vi "Process.vi"(8 "error in":errorcluster, 11 "Example Instrument UI":refnum<class "Instrument.Example UI.lvclass">) -> (0 "error out":errorcluster, 3 "Example Instrument UI out":refnum<class "Instrument.Example UI.lvclass">)   [LabVIEW 2016, in "Instrument.Example UI.lvclass"]
doc: "---------------------------------------------------------------\nJKI State Machine Objects™\nhttp://jki.net/state-machine-objects/\nCopyright (C) 2005-2015, JKI <info@jki.net>\nALL RIGHTS RESERVEDJKI State Machine Objects (SMO) 1.0.0.5\nJKI - JKI\nCopyright (c) 2016, JKI"
uses:
  Instrument.Example UI.lvclass
  C:/Program Files (x86)/National Instruments/LabVIEW 2016/vi.lib/JKI/JKI SMO/SMO/SMO.lvclass
  C:/Program Files (x86)/National Instruments/LabVIEW 2016/vi.lib/JKI/JKI SMO/SMO.UI/SMO.UI.lvclass
  <vilib>/JKI/JKI SMO/SMO/Typedefs/Parent Call--Enum.ctl
  Instrument.Example UI.lvclass/Instrument.Example UI.ctl
  <vilib>/JKI/JKI SMO/SMO.UI/SMO.UI.lvclass
  <vilib>/JKI/JKI SMO/SMO/SMO.lvclass
  <userlib>/LevyLab/Levylab Instruments/SMOs/Instrument/Instrument.lvclass
panel:
  in  "setConfig":bool
  in  "update time (ms)":u32=200
  in  "STOP":bool
  # "#todo\nmake UI here. maybe include a nice picture of the hardware?\n#todo\nadd buttons to do stuff (e.g., change a setting)\nButtons should trigger an event\n#todo\nresize this box if you want your UI to be different size"
  # "#todo\nthis control is refresh rate"
  # "SMO UI Template"
  # "For instructions on how to use the JKI State Machine Objects, examples and video tutorials, visit:\nhttp://jki.net/state-machine-objects/\n\nJKI State Machine Objects™\nhttp://jki.net/state-machine-objects/\nCopyright (C) 2005-2015, JKI <info@jki.net>\nALL RIGHTS RESERVED"
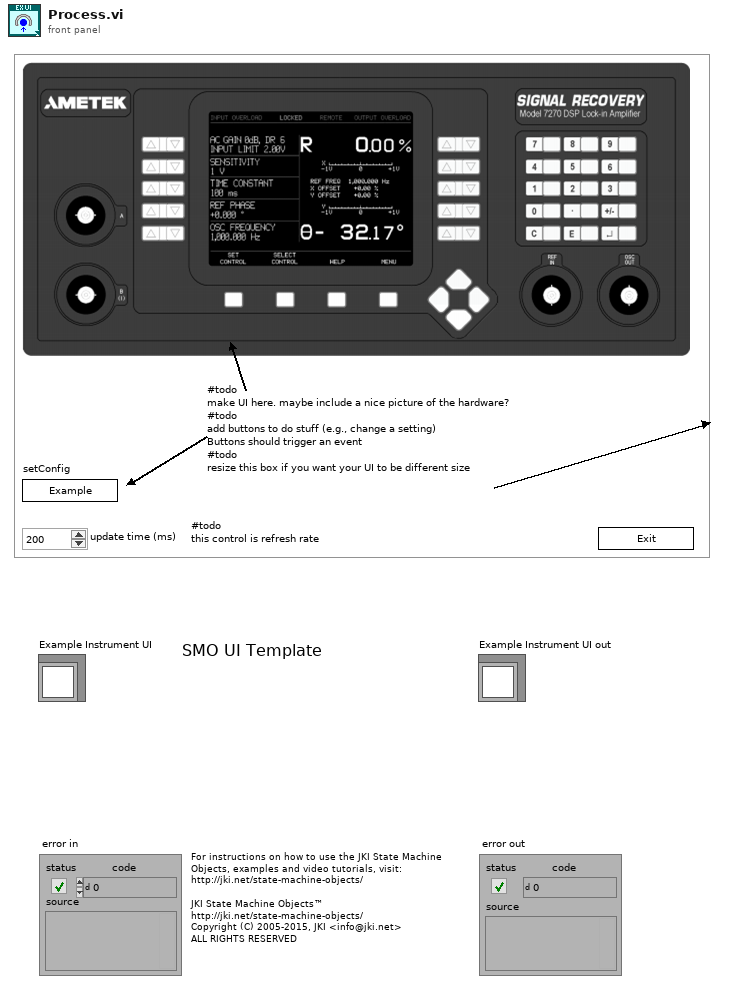
[diagram p1: front panel]
types:
  T1 = typedef "SMO.lvclass/Parent Call--Enum.ctl" = enum16{"Allows parent to run", "Does not request parent to run"}
  T2 = enum32{"invalid app kind", "Development System", "Run Time System", "Student Edition", "Embedded LabVIEW", "Evaluation", "Custom"}
  T3 = enum32{"Invalid", "Standard", "Closed", "Hidden", "Minimized", "Maximized"}
  T4 = cluster{"Core":cluster{"Current VI Reference":refnum<vi>, "Close Panel on Exit?":bool, "error":errorcluster}, "Self Reference":refnum<class "Instrument.Example UI.lvclass">, "Instrument":refnum<class "Instrument.lvclass">, "getAll":variant, "getDisplay":variant, "config":variant}
  T5 = cluster{"Current VI Reference":refnum<vi>, "Close Panel on Exit?":bool, "error":errorcluster}
  T6 = typedef "SMO.lvclass/Protected Events.ctl" = cluster{"StopProcesses":refnum<user-event>, "AbortProcesses":refnum<user-event>, "Config Changed":refnum<user-event>, "Dependency":refnum<user-event>}
  T7 = typedef "Instrument.lvclass/PublicEvents--Cluster.ctl" = cluster{"MessageFromProcess":refnum<user-event>}
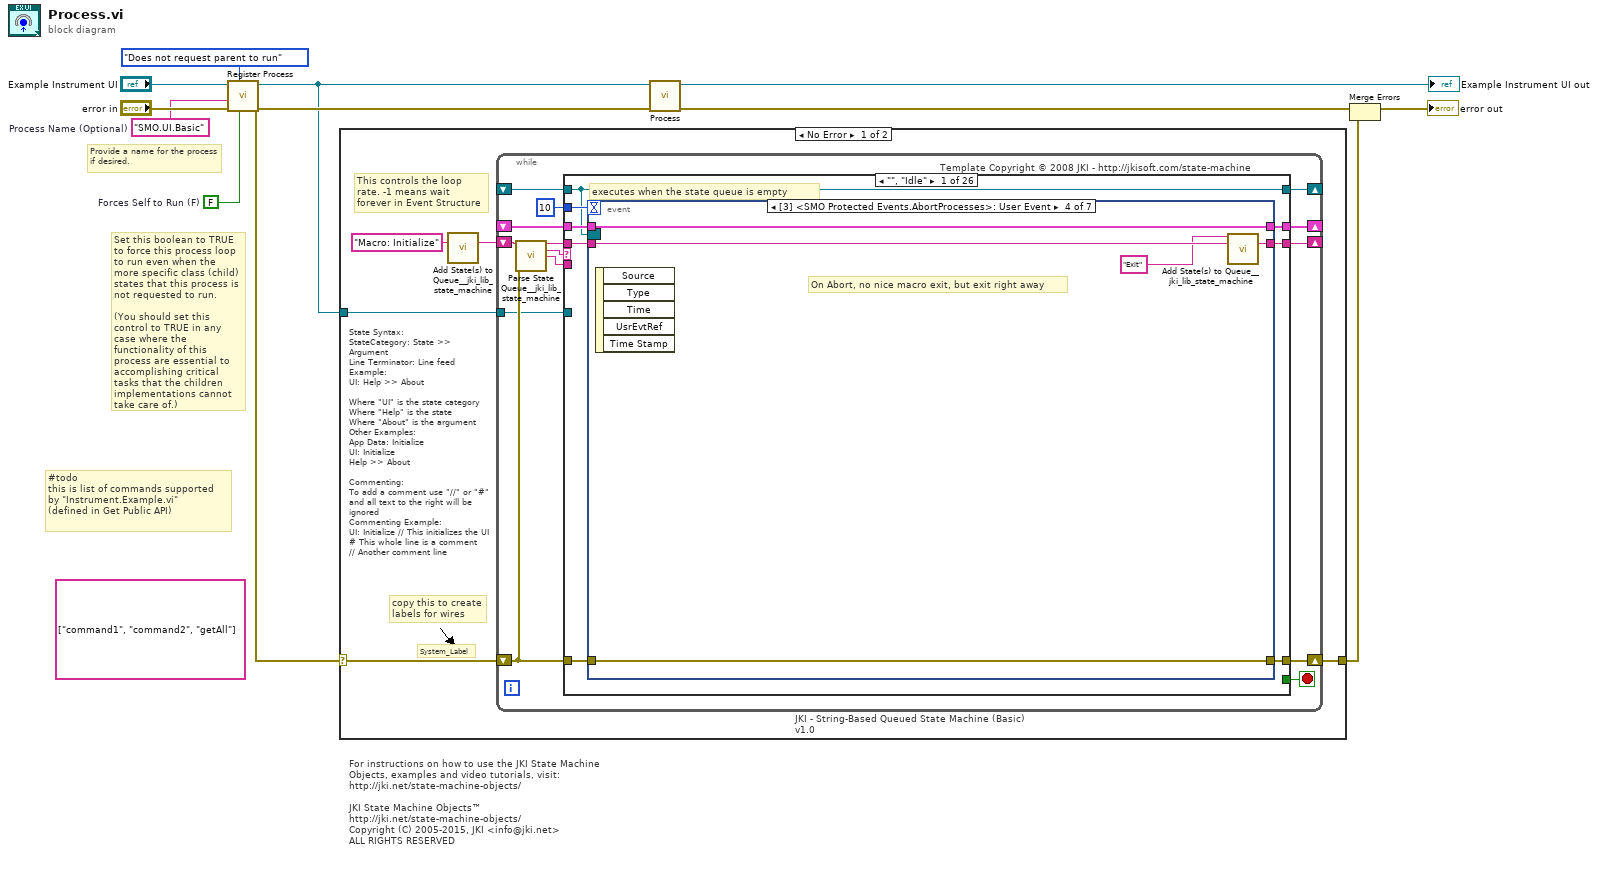
[diagram p0: block diagram]
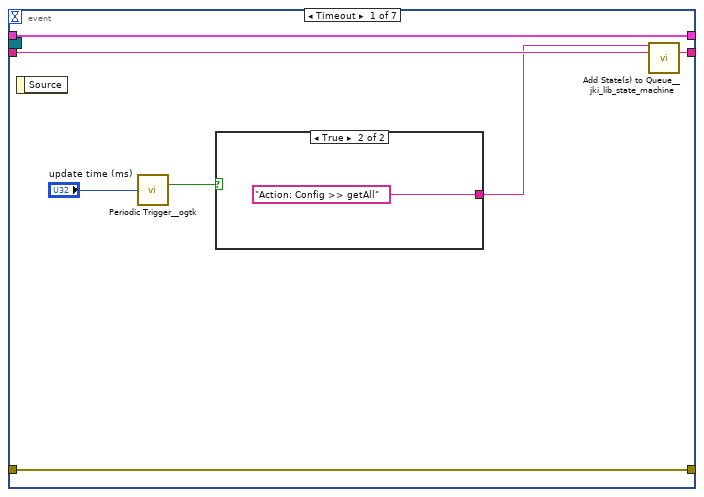
[diagram p2: hidden frame]
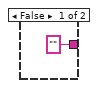
[diagram p3: hidden frame]
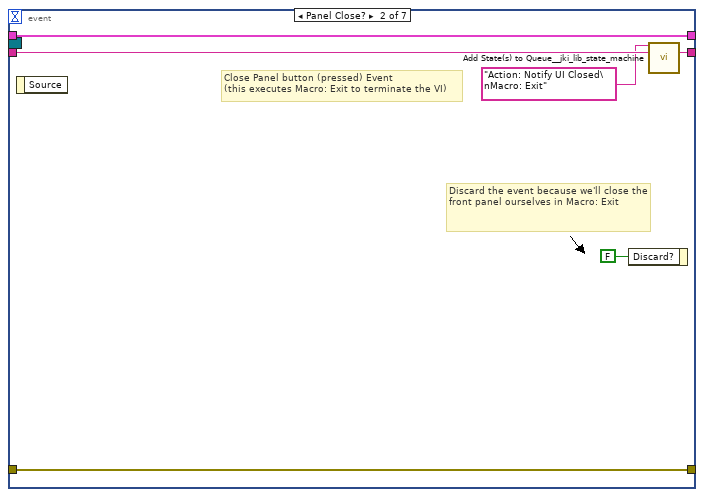
[diagram p4: hidden frame]
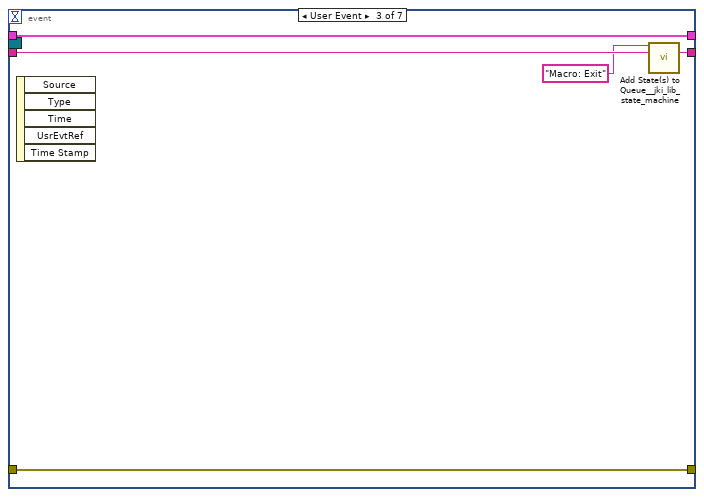
[diagram p5: hidden frame]
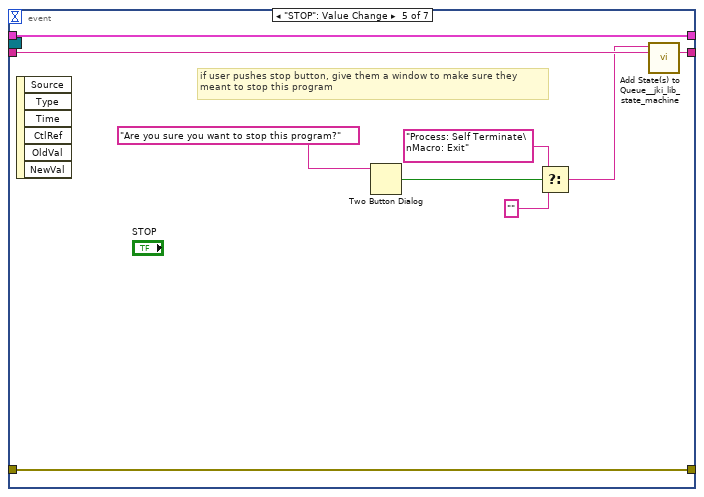
[diagram p6: hidden frame]
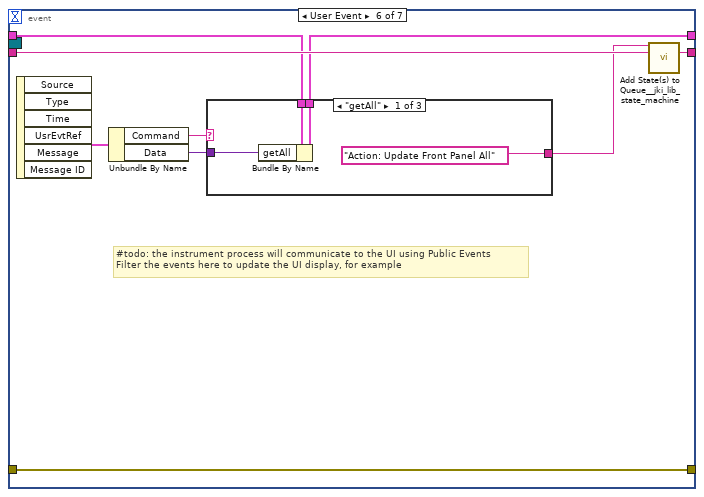
[diagram p7: hidden frame]
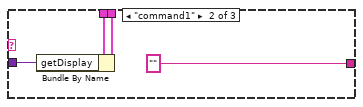
[diagram p8: hidden frame]
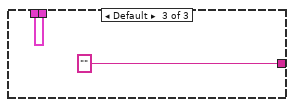
[diagram p9: hidden frame]
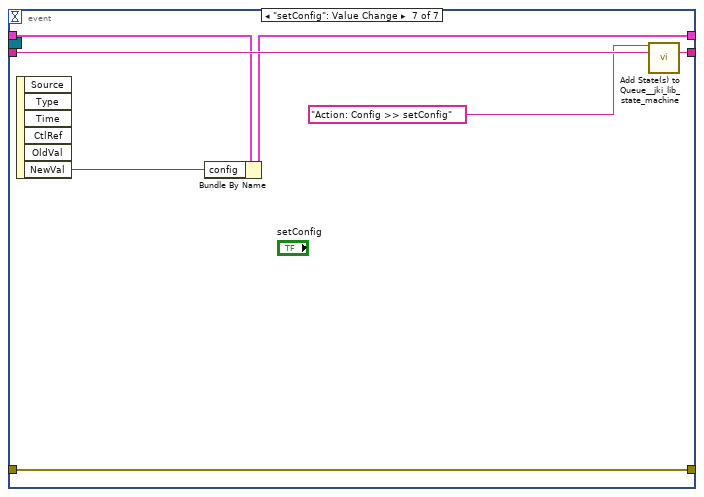
[diagram p10: hidden frame]
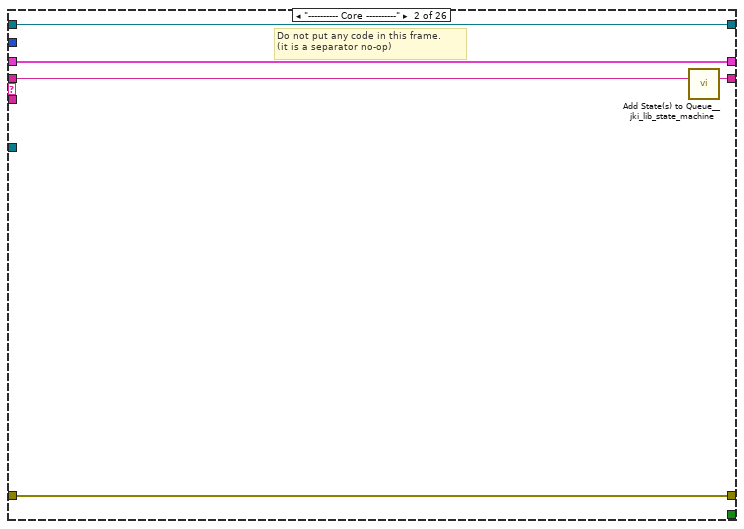
[diagram p11: hidden frame]
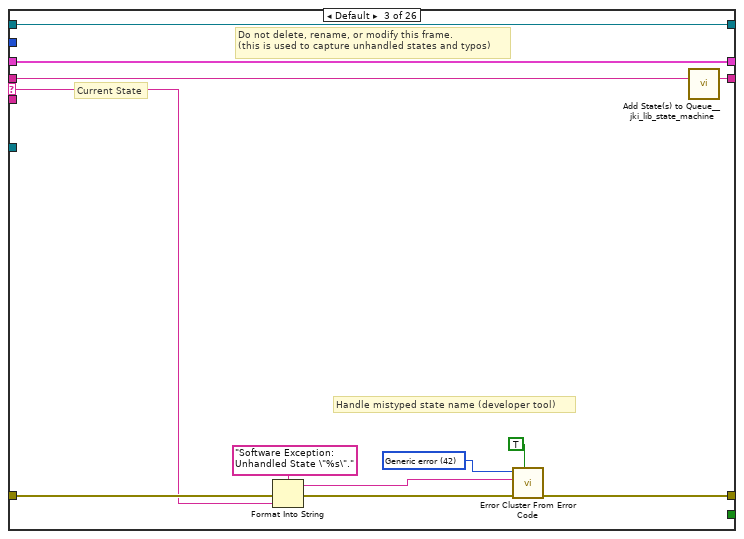
[diagram p12: hidden frame]
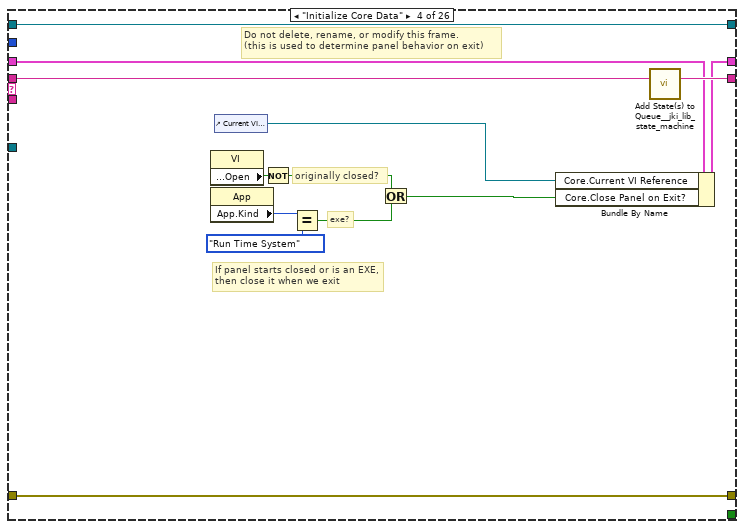
[diagram p13: hidden frame]
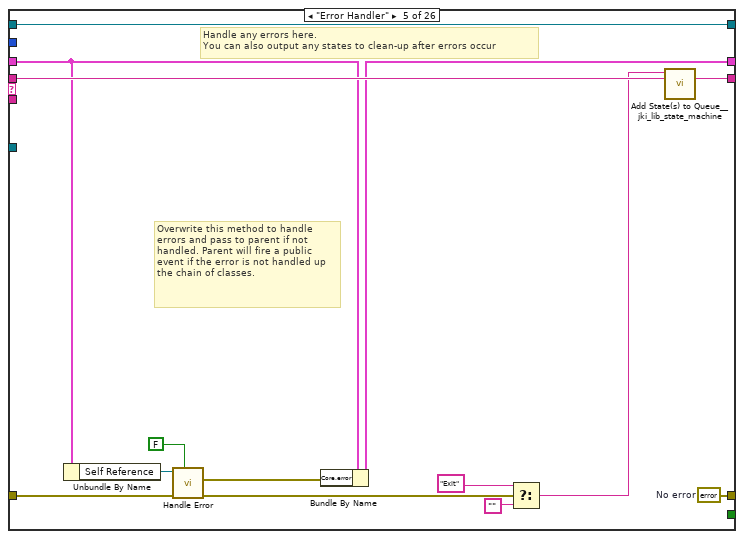
[diagram p14: hidden frame]
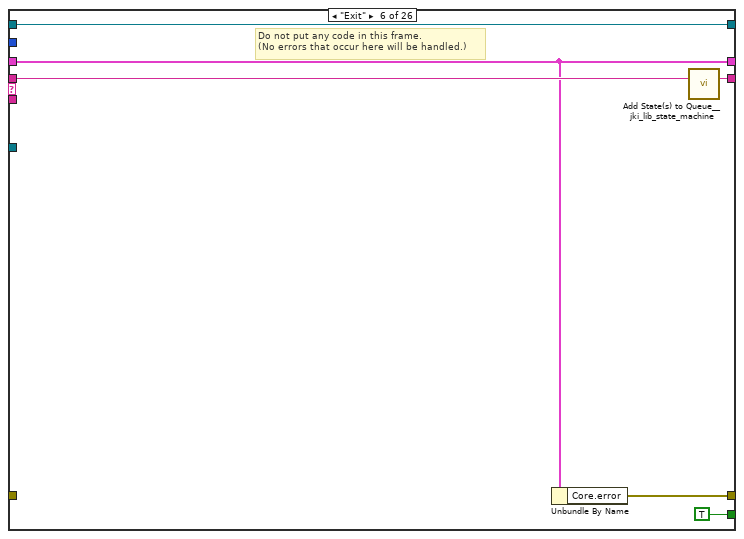
[diagram p15: hidden frame]
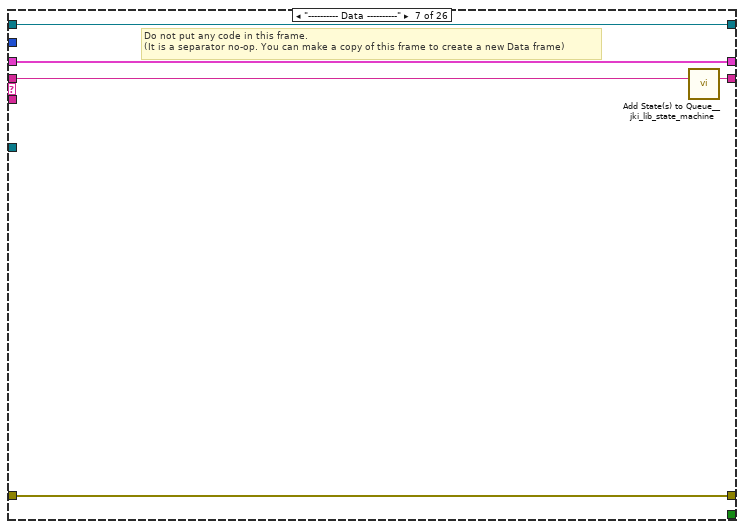
[diagram p16: hidden frame]
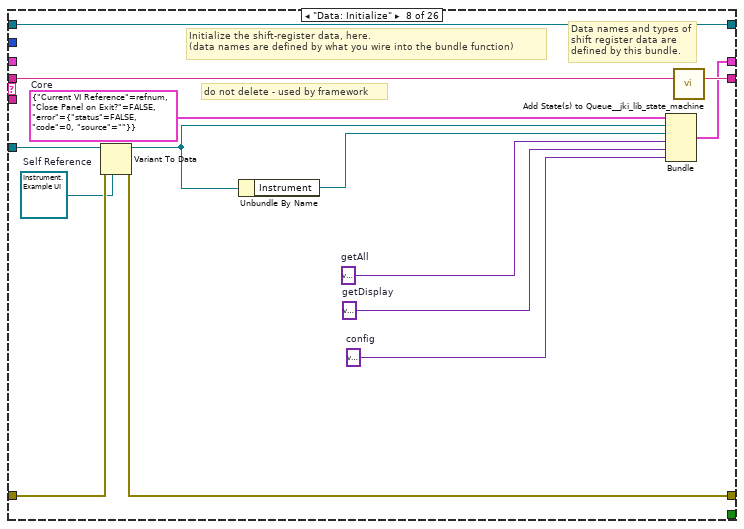
[diagram p17: hidden frame]
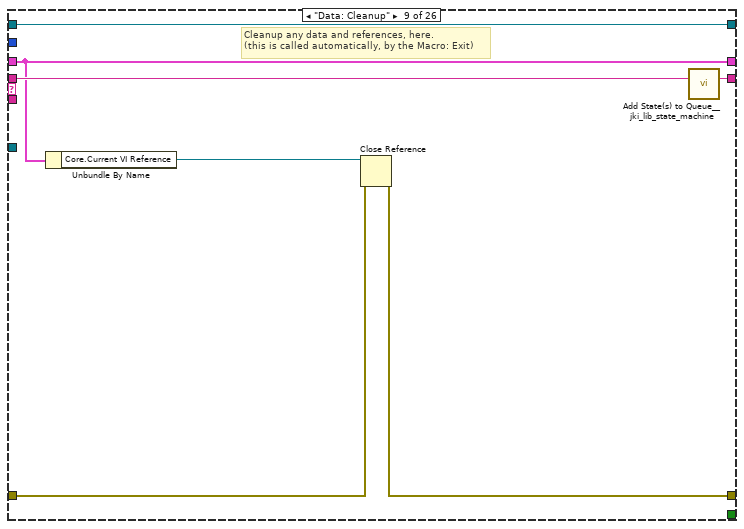
[diagram p18: hidden frame]
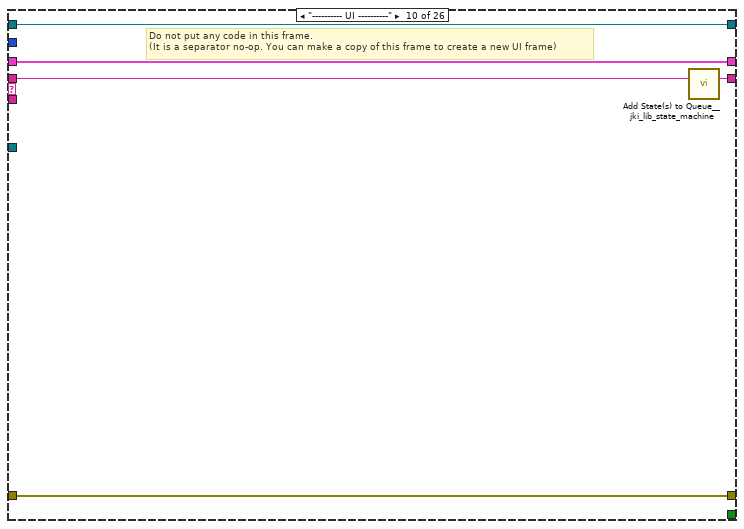
[diagram p19: hidden frame]
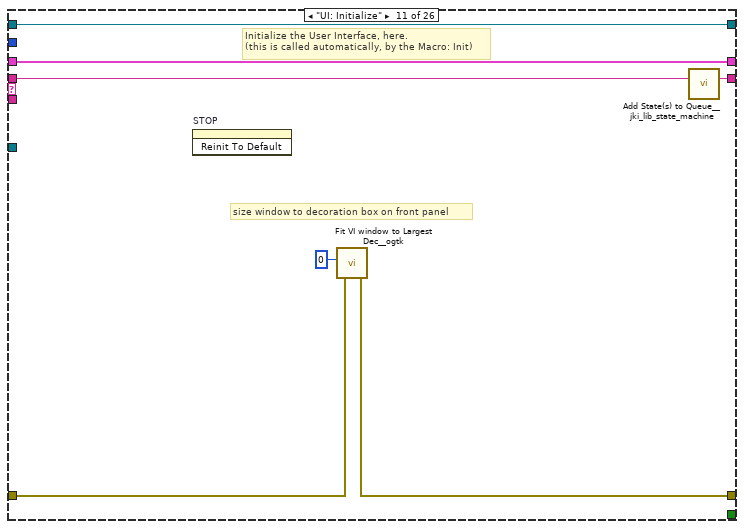
[diagram p20: hidden frame]
diagram:
  (unwired) string[] ["command1", "command2", "getAll"] ("element")
  w2 = FALSE  # Forces Self to Run (F)
  w1 = "SMO.UI.Basic"  # Process Name (Optional)
  # "#todo\nthis is list of commands supported\nby \"Instrument.Example.vi\"\n(defined in Get Public API)"
  # "Provide a name for the process\nif desired."
  # "Set this boolean to TRUE to force this process loop to run even when the more specific class (child) states that this process is not requested to run.\n\n(You should set this control to TRUE in any case where the functionality of this process are essential to accomplishing critical tasks that the children implementations cannot take care of.)"
  # "For instructions on how to use the JKI State Machine Objects, examples and video tutorials, visit:\nhttp://jki.net/state-machine-objects/\n\nJKI State Machine Objects™\nhttp://jki.net/state-machine-objects/\nCopyright (C) 2005-2015, JKI <info@jki.net>\nALL RIGHTS RESERVED"
  n1 = call <vilib>:"Register Process.vi"("Forces Self to Run (F)"=w2, "Parent Call"=Parent_Call--Enum."Does not request parent to run", "error in (no error)"="error in", "Process Name (optional)"=w1, "SMO"="Example Instrument UI") -> ("error out"=w8:errorcluster, "SMO out"=w7:refnum<class "Instrument.Example UI.lvclass">)  [unwired: 5 in]
  n2 = case shown="No Error" w8 {
    selector: w8 -> [w13 w343]
    tunnel: w7 -> [w14 _]
    tunnel: [w12 w343] -> w4
    frame No Error {
      # "State Syntax:\nStateCategory: State >> Argument\nLine Terminator: Line feed\nExample:\nUI: Help >> About\n\nWhere \"UI\" is the state category\nWhere \"Help\" is the state\nWhere \"About\" is the argument\nOther Examples:\nApp Data: Initialize\nUI: Initialize\nHelp >> About\n\nCommenting:\nTo add a comment use \"//\" or \"#\" and all text to the right will be ignored\nCommenting Example:\nUI: Initialize // This initializes the UI\n# This whole line is a comment\n// Another comment line"
      # "copy this to create labels for wires"
      # "This controls the loop rate. -1 means wait forever in Event Structure"
      # "System_Label"
      n3 = call <vilib>:"Add State(s) to Queue__jki_lib_state_machine.vi"("State(s) in (\"\")"="Macro: Initialize") -> ("States Out"=w16:string)  [unwired: 14 in]
      n4 = while "JKI - String-Based Queued State Machine (Basic) v1.0" {
        shift-right: [w23] -> _
        shift-left: _ -> [w22]
        shift-right: [w26] -> w12
        shift-left: w13 -> [w20]
        shift-right: [w25] -> _
        shift-left: w16 -> [w27]
        tunnel: w14 -> [w19]
        shift-right: [w18] -> _
        shift-left: _ -> [w17]
        stop <- w24 stop-if-true
        # "Template Copyright © 2008 JKI - http://jkisoft.com/state-machine"
        n5 = call <vilib>:"Parse State Queue__jki_lib_state_machine.vi"("State Queue"=w27, "Error In (no error)"=w20) -> ("Remaining States"=w29:string, "Current State"=w30:string, "Arguments"=w28:string)  [unwired: 11 in]
        n6 = case shown="\"\", \"Idle\"" w30 {
          selector: w30 -> [_ _ w105 _ _ _ _ _ _ _ _ _ _ _ _ _ _ _ _ _ _ _ _ _ _ _]
          tunnel: w29 -> [w38 w103 w109 w128 w142 w148 w153 w167 w174 w179 w186 w193 w209 w241 w250 w264 w269 w280 w287 w292 w305 w311 w318 w325 w333 w342]
          tunnel: w28 -> [_ _ _ _ _ _ _ _ _ _ _ w187 w203 _ _ _ _ _ _ _ _ _ _ _ _ w334]
          tunnel: w22 -> [w36 w100 w107 w119 w130 w144 w150 _ w169 w176 w184 w191 w205 w238 w246 w255 w266 w277 w282 w289 w303 w309 w314 w321 w330 w339]
          tunnel: [w35 w101 w111 w125 w135 w143 w151 w163 w170 w177 w181 w188 w206 w239 w248 w262 w267 w271 w283 w290 w298 w306 w315 w319 w328 w337] -> w26
          tunnel: w20 -> [w34 w101 w110 w125 w131 _ w151 w164 w171 w177 w182 w189 w207 w239 w248 w262 w267 w272 w284 w290 w300 w307 w315 w320 w329 w335]
          tunnel: [w37 w102 w108 w127 w141 w147 w152 w166 w173 w178 w185 w192 w208 w240 w249 w263 w268 w279 w286 w291 w304 w310 w317 w324 w332 w341] -> w25
          tunnel: [_ _ _ _ _ TRUE _ _ _ _ _ _ _ _ _ _ _ _ _ _ _ _ _ _ _ _] -> w24
          tunnel: [w33 w100 w107 w126 w133 w144 w150 w165 w169 w176 w184 w191 w205 w238 w246 w255 w266 w277 w282 w289 w303 w309 w313 w321 w330 w339] -> w23
          tunnel: 10 ("Timeout") -> [w32 _ _ _ _ _ _ _ _ _ _ _ _ _ _ _ _ _ _ _ _ _ _ _ _ _]
          tunnel: w19 -> [_ _ _ _ _ _ _ w161 _ _ _ _ _ _ _ _ _ _ _ _ _ _ _ _ _ _]
          tunnel: [w31 w99 w104 w116 w140 w145 w149 w160 w168 w175 w183 w190 w202 w237 w247 w256 w265 w278 w285 w288 w302 w308 w316 w323 w331 w340] -> w18
          tunnel: w17 -> [w31 w99 w104 w116 w140 w145 w149 w160 w168 w175 w183 w190 w202 w237 w247 w256 w265 w278 w285 w288 _ w308 w316 w323 w331 w340]
          frame "", "Idle" {
            # "executes when the state queue is empty"
            n7 = event shown="[3] <SMO Protected Events.AbortProcesses>: User Event" {
              selector: w31 -> [_ _ _ _ _ _ _]
              dyn-events: _ -> [_ _ _ _ _ _ _]
              timeout: w32 -> [_ _ _ _ _ _ _]
              tunnel: w38 -> [w45 w53 w58 w63 w72 w81 w98]
              tunnel: [w44 w52 w57 w62 w71 w80 w97] -> w37
              tunnel: w36 -> [w42 w49 w55 w60 w69 w77 w94]
              tunnel: [w43 w48 w56 w61 w70 w79 w95] -> w35
              tunnel: w34 -> [w43 w48 w56 w61 w70 w79 w95]
              tunnel: [w42 w49 w55 w60 w69 w76 w93] -> w33
              event Timeout {
                n8 = event-data() -> ()  [unwired: 1 in, 1 out]
                n9 = call <userlib>:"Periodic Trigger__ogtk.vi"("time (ms)"="update time (ms)") -> ("Triggered"=w41:bool)  [unwired: 12 in, 2 out]
                n10 = case shown="True" w41 {
                  tunnel: ["" "Action: Config >> getAll"] -> w39
                  frame False {
                  }
                  frame True {
                  }
                }
                n11 = call <vilib>:"Add State(s) to Queue__jki_lib_state_machine.vi"("State(s) in Front (\"\")"=w39, "State(s) in (\"\")"=w45) -> ("States Out"=w44:string)  [unwired: 13 in]
              }
              event Panel Close? {
                # "Discard the event because we'll close the front panel ourselves in Macro: Exit"
                # "Close Panel button (pressed) Event\n(this executes Macro: Exit to terminate the VI)"
                n12 = event-data() -> ()  [unwired: 1 in, 1 out]
                n13 = event-data("Discard?"=FALSE) -> ()  [unwired: 1 in, 1 out]
                n14 = call <vilib>:"Add State(s) to Queue__jki_lib_state_machine.vi"("State(s) in Front (\"\")"="Action: Notify UI Closed\nMacro: Exit", "State(s) in (\"\")"=w53) -> ("States Out"=w52:string)  [unwired: 13 in]
              }
              event User Event {
                n15 = event-data() -> ()  [unwired: 1 in, 5 out]
                n16 = call <vilib>:"Add State(s) to Queue__jki_lib_state_machine.vi"("State(s) in Front (\"\")"="Macro: Exit", "State(s) in (\"\")"=w58) -> ("States Out"=w57:string)  [unwired: 13 in]
              }
              event User Event {
                # "On Abort, no nice macro exit, but exit right away"
                n17 = event-data() -> ()  [unwired: 1 in, 5 out]
                n18 = call <vilib>:"Add State(s) to Queue__jki_lib_state_machine.vi"("State(s) in Front (\"\")"="Exit", "State(s) in (\"\")"=w63) -> ("States Out"=w62:string)  [unwired: 13 in]
              }
              event "STOP": Value Change {
                # "if user pushes stop button, give them a window to make sure they\nmeant to stop this program"
                n19 = event-data() -> ()  [unwired: 1 in, 6 out]
                n20 = Two Button Dialog(message="Are you sure you want to stop this program?") -> (T button?=w68:bool)  [unwired: 2 in]
                n21 = Select(t="Process: Self Terminate\nMacro: Exit", s=w68, f="") -> (s? t:f=w64:string)
                n22 = call <vilib>:"Add State(s) to Queue__jki_lib_state_machine.vi"("State(s) in Front (\"\")"=w64, "State(s) in (\"\")"=w72) -> ("States Out"=w71:string)  [unwired: 13 in]
              }
              event User Event {
                # "#todo: the instrument process will communicate to the UI using Public Events\nFilter the events here to update the UI display, for example"
                n23 = event-data() -> ("Message"=w78:cluster{"Command":string, "Data":variant})  [unwired: 1 in, 5 out]
                n24 = Unbundle By Name(w78) -> ("Command"=w74:string, "Data"=w75:variant)
                n25 = case shown="\"getAll\"" w74 {
                  tunnel: w75 -> [w85 w89 _]
                  tunnel: w77 -> [w84 w88 w90]
                  tunnel: [w83 w87 w90] -> w76
                  tunnel: ["Action: Update Front Panel All" "" ""] -> w73
                  frame "getAll" {
                    n26 = Bundle By Name(cluster=w84, "getAll"=w85) -> (w83:T4)
                  }
                  frame "command1" {
                    n27 = Bundle By Name(cluster=w88, "getDisplay"=w89) -> (w87:T4)
                  }
                  frame Default {
                  }
                }
                n28 = call <vilib>:"Add State(s) to Queue__jki_lib_state_machine.vi"("State(s) in Front (\"\")"=w73, "State(s) in (\"\")"=w81) -> ("States Out"=w80:string)  [unwired: 13 in]
              }
              event "setConfig": Value Change {
                n29 = event-data() -> ("NewVal"=w92:bool)  [unwired: 1 in, 5 out]
                n30 = Bundle By Name(cluster=w94, "config"=w92) -> (w93:T4)
                n31 = call <vilib>:"Add State(s) to Queue__jki_lib_state_machine.vi"("State(s) in Front (\"\")"="Action: Config >> setConfig", "State(s) in (\"\")"=w98) -> ("States Out"=w97:string)  [unwired: 13 in]
              }
            }
          }
          frame "---------- Core ----------" {
            # "Do not put any code in this frame.\n(it is a separator no-op)"
            n32 = call <vilib>:"Add State(s) to Queue__jki_lib_state_machine.vi"("State(s) in (\"\")"=w103) -> ("States Out"=w102:string)  [unwired: 14 in]
          }
          frame Default {
            w114 = 42 items=["No error", "Argument error", "Memory is full", "Out of zone", "End of file", "File already open", "Generic file I/O error", "File not found", "File permission error", "Disk is full", "Duplicate path", "Too many files open", "System feature not enabled", "Resource file not found", "Cannot add resource", "Resource not found", "Image not found", "Image memory error", "Pen does not exist", "Config type invalid", "Config token not found", "Config parse error", "Config memory error", "Bad external code format", "Bad external code offset", "External code not present", "Null window", "Destroy window error", "Null menu", "Print aborted", "Bad print record", "Print driver error", "Windows error during printing", "Memory error during printing", "Print dialog error", "Generic print error", "Invalid device refnum", "Device not found", "Device parameter error", "Device unit error", "Cannot open device", "Device call aborted", "Generic error", "Cancelled by user", "Object ID too low", "Object ID too high", "Object not in heap", "Unknown heap", "Unknown object (invalid DefProc)", "Unknown object (DefProc not in table)", "Message out of range", "Invalid (null) method", "Unknown message", "Manager call not supported", "Bad address", "Network operation in progress", "Network operation timed out", "Connection is busy", "Network attribute not supported", "Network error", "Address in use", "System out of memory", "Connection aborted", "Connection refused", "Not connected", "Already connected", "Connection closed", "Initialization error (interapplication manager)", "Bad occurrence", "Wait on unbound occurrence handler", "Occurrence queue overflow", "Datalog type conflict", "Unused", "Unrecognized type (interapplication manager)", "Memory corrupt", "Failed to make temporary DLL", "Old CIN version", "Drag socket not found", "Failed to load drop-object", "Failed to register OLE object", "Failed to release OLE object", "Format specifier type mismatch", "Unknown format specifier", "Too few format specifiers", "Too many format specifiers", "Scan failed", "Newer CIN version", "Error converting to variant", "Runtime menu error", "Password tampered", "Variant attribute not found", "Incompatible variant data type", "Event data is not available", "Event Store is not present", "Occurrence is not found", "Event Queue is not created", "Event info is not available", "Refnum passed is NULL", "Error retrieving Class GUID", "Error retrieving CoClass GUID", "Error retrieving TypeLib GUID.", "Bad built application magic bytes.", "Specific driver is different from the specific driver associated with the Logical Name.", "There is no session opened to the class driver.", "Max Error", "MAX - Error with config objects", "MAX - Error loading configuration", "MAX - Group not supported"]
            # "Current State"
            # "Do not delete, rename, or modify this frame.\n(this is used to capture unhandled states and typos)"
            # "Handle mistyped state name (developer tool)"
            n33 = Format Into String(format string="Software Exception: Unhandled State \"%s\"." ("message"), error in=w110, w105) -> (resulting string=w113:string, error out=w112:errorcluster)  [unwired: 1 in]
            n34 = call <vilib>:"Error Cluster From Error Code.vi"("show call chain? (False)"=TRUE, "error in (no error)"=w112, "error message (\"\")"=w113, "error code (0)"=w114) -> ("error out"=w111:errorcluster)  [unwired: 5 in]
            n35 = call <vilib>:"Add State(s) to Queue__jki_lib_state_machine.vi"("State(s) in (\"\")"=w109) -> ("States Out"=w108:string)  [unwired: 14 in]
          }
          frame "Initialize Core Data" {
            # "Do not delete, rename, or modify this frame.\n(this is used to determine panel behavior on exit)"
            # "originally closed?"
            # "exe?"
            # "If panel starts closed or is an EXE, then close it when we exit"
            n36 = property class="VI"() -> ("Front Panel.Open"=w124:bool)  [unwired: 2 in, 2 out]
            n37 = property class="App"() -> ("App.Kind"=w123:T2)  [unwired: 2 in, 2 out]
            n38 = control-ref of="Current VI Reference"() -> (w117:refnum<vi>)
            n39 = Not(x=w124) -> (.not. x?=w121:bool)
            n40 = Equal?(x=w123, y=T2."Run Time System" ("Application:Kind")) -> (x = y?=w120:bool)
            n41 = Or(x=w121, y=w120) -> (x .or. y?=w118:bool)
            n42 = Bundle By Name(cluster=w119, "Core.Current VI Reference"=w117, "Core.Close Panel on Exit?"=w118) -> (w126:T4)
            n43 = call <vilib>:"Add State(s) to Queue__jki_lib_state_machine.vi"("State(s) in (\"\")"=w128) -> ("States Out"=w127:string)  [unwired: 14 in]
          }
          frame "Error Handler" {
            w135 = errorcluster {"status"=FALSE, "code"=0, "source"=""}  # No error
            # "Overwrite this method to handle errors and pass to parent if not handled. Parent will fire a public event if the error is not handled up the chain of classes."
            # "Handle any errors here.\nYou can also output any states to clean-up after errors occur"
            n44 = Unbundle By Name(w130) -> ("Self Reference"=w139:refnum<class "Instrument.Example UI.lvclass">)
            n45 = call-dynamic "Handle Error.vi"("Stop on Unhandled Error (T)"=FALSE, "error in"=w131, "SMO"=w139) -> ("handling error"=w129:errorcluster, "Unhandled error"=w134:errorcluster)  [unwired: 6 in, 1 out]
            n46 = Bundle By Name(cluster=w130, "Core.error"=w134) -> (w133:T4)
            n47 = Select(t="Exit", s=w129, f="") -> (s? t:f=w136:string)
            n48 = call <vilib>:"Add State(s) to Queue__jki_lib_state_machine.vi"("State(s) in Front (\"\")"=w136, "State(s) in (\"\")"=w142) -> ("States Out"=w141:string)  [unwired: 13 in]
          }
          frame "Exit" {
            # "Do not put any code in this frame.\n(No errors that occur here will be handled.)"
            n49 = Unbundle By Name(w144) -> ("Core.error"=w143:errorcluster)
            n50 = call <vilib>:"Add State(s) to Queue__jki_lib_state_machine.vi"("State(s) in (\"\")"=w148) -> ("States Out"=w147:string)  [unwired: 14 in]
          }
          frame "---------- Data ----------" {
            # "Do not put any code in this frame.\n(It is a separator no-op. You can make a copy of this frame to create a new Data frame)"
            n51 = call <vilib>:"Add State(s) to Queue__jki_lib_state_machine.vi"("State(s) in (\"\")"=w153) -> ("States Out"=w152:string)  [unwired: 14 in]
          }
          frame "Data: Initialize" {
            w154 = variant  # config
            w155 = variant  # getDisplay
            w156 = variant  # getAll
            w159 = T5 {"Current VI Reference"=refnum, "Close Panel on Exit?"=FALSE, "error"={"status"=FALSE, "code"=0, "source"=""}}  # Core
            w162 = refnum<class "Instrument.Example UI.lvclass"> refnum  # Self Reference
            # "do not delete - used by framework"
            # "Data names and types of shift register data are defined by this bundle."
            # "Initialize the shift-register data, here.\n(data names are defined by what you wire into the bundle function)"
            n52 = Variant To Data(error in=w164, type=w162, Variant=w161) -> (data=w158:refnum<class "Instrument.Example UI.lvclass">, error out=w163:errorcluster)
            n53 = Unbundle By Name(w158) -> ("Instrument"=w157:refnum<class "Instrument.lvclass">)
            n54 = Bundle("Core"=w159, "Self Reference"=w158, "Instrument"=w157, "getAll"=w156, "getDisplay"=w155, "config"=w154) -> (w165:T4)  [unwired: 1 in]
            n55 = call <vilib>:"Add State(s) to Queue__jki_lib_state_machine.vi"("State(s) in (\"\")"=w167) -> ("States Out"=w166:string)  [unwired: 14 in]
          }
          frame "Data: Cleanup" {
            # "Cleanup any data and references, here.\n(this is called automatically, by the Macro: Exit)"
            n56 = Unbundle By Name(w169) -> ("Core.Current VI Reference"=w172:refnum<vi>)
            n57 = Close Reference(reference=w172, error in (no error)=w171) -> (error out=w170:errorcluster)
            n58 = call <vilib>:"Add State(s) to Queue__jki_lib_state_machine.vi"("State(s) in (\"\")"=w174) -> ("States Out"=w173:string)  [unwired: 14 in]
          }
          frame "---------- UI ----------" {
            # "Do not put any code in this frame.\n(It is a separator no-op. You can make a copy of this frame to create a new UI frame)"
            n59 = call <vilib>:"Add State(s) to Queue__jki_lib_state_machine.vi"("State(s) in (\"\")"=w179) -> ("States Out"=w178:string)  [unwired: 14 in]
          }
          frame "UI: Initialize" {
            # "size window to decoration box on front panel"
            # "Initialize the User Interface, here.\n(this is called automatically, by the Macro: Init)"
            n60 = invoke on="STOP" class="Bool (strict)" method="Reinit To Default"() -> ()  [unwired: 3 in, 3 out]
            n61 = call <userlib>:"Fit VI window to Largest Dec__ogtk.vi"("error in (no error)"=w182, "border spacing (2 px)"=0) -> ("error out"=w181:errorcluster)  [unwired: 4 in, 1 out]
            n62 = call <vilib>:"Add State(s) to Queue__jki_lib_state_machine.vi"("State(s) in (\"\")"=w186) -> ("States Out"=w185:string)  [unwired: 14 in]
          }
          frame "UI: Cursor Set" {
            # "Argument"
            # "Initialize the User Interface, here.\n(this is called automatically, by the Macro: Init)"
            n63 = disable-structure shown="Default" {
              disable-tunnel: w189 -> [w194 w197]
              disable-tunnel: [w194 w196] -> w188
              disable-tunnel: w187 -> [_ w195]
              frame condition #0 {
              }
              frame condition #1 (active) {
                n64 = case shown="\"Busy\"" w195 {
                  tunnel: w197 -> [w199 w201]
                  tunnel: [w198 w200] -> w196
                  frame "Idle", Default {
                    n65 = call <vilib>:"Unset Busy.vi"("error in (no error)"=w199) -> ("error out"=w198:errorcluster)  [unwired: 10 in]
                  }
                  frame "Busy" {
                    n66 = call <vilib>:"Set Busy.vi"("error in (no error)"=w201) -> ("error out"=w200:errorcluster)  [unwired: 9 in, 1 out]
                  }
                }
              }
            }
            n67 = call <vilib>:"Add State(s) to Queue__jki_lib_state_machine.vi"("State(s) in (\"\")"=w193) -> ("States Out"=w192:string)  [unwired: 14 in]
          }
          frame "UI: Front Panel State" {
            # "Argument"
            # "Set Front Panel Open or Closed\n(Usage: \"UI: Front Panel State >> Open|Close\")"
            n68 = Unbundle By Name(w205) -> ("Core.Current VI Reference"=w204:refnum<vi>)
            n69 = disable-structure shown="Default" {
              disable-tunnel: w207 -> [w213 w236]
              disable-tunnel: [w212 w236] -> w206
              disable-tunnel: w204 -> [w211 _]
              disable-tunnel: w203 -> [w210 _]
              frame condition #0 (active) {
                n70 = case shown="\"Close\"" w210 {
                  tunnel: w213 -> [w217 w230]
                  tunnel: [w219 w231] -> w212
                  tunnel: w211 -> [w218 w228]
                  frame "Open", Default {
                    n71 = property class="VI"(reference=w218, error in=w217) -> (reference out=w215:refnum<vi>, error out=w216:errorcluster, "FP.State"=w214:T3)
                    n72 = case shown="\"Closed\"" w214 {
                      tunnel: [w222 w225] -> w219
                      tunnel: w216 -> [w221 w225]
                      tunnel: w215 -> [w220 _]
                      frame "Closed" {
                        n73 = invoke class="VI" method="FP.Open"(reference=w220, error in=w221, "Activate"=TRUE, "State"=T3."Standard") -> (error out=w222:errorcluster)  [unwired: 1 in, 4 out]
                      }
                      frame Default {
                      }
                    }
                  }
                  frame "Close" {
                    n74 = property class="VI"(reference=w228, error in=w230) -> (reference out=w227:refnum<vi>, error out=w229:errorcluster, "FP.State"=w226:T3)
                    n75 = case shown="Default" w226 {
                      tunnel: [w232 w235] -> w231
                      tunnel: w229 -> [w232 w234]
                      tunnel: w227 -> [_ w233]
                      frame "Invalid", "Closed" {
                      }
                      frame Default {
                        n76 = invoke class="VI" method="FP.Close"(reference=w233, error in=w234) -> (error out=w235:errorcluster)  [unwired: 1 in, 2 out]
                      }
                    }
                  }
                }
              }
              frame condition #1 {
              }
            }
            n77 = call <vilib>:"Add State(s) to Queue__jki_lib_state_machine.vi"("State(s) in (\"\")"=w209) -> ("States Out"=w208:string)  [unwired: 14 in]
          }
          frame "---------- Macro ----------" {
            # "Do not put any code in this frame.\n(It is a separator no-op. You can make a copy of this frame to create a new Macro frame)"
            n78 = call <vilib>:"Add State(s) to Queue__jki_lib_state_machine.vi"("State(s) in (\"\")"=w241) -> ("States Out"=w240:string)  [unwired: 14 in]
          }
          frame "Macro: Initialize" {
            w244 = "UI: Initialize\nUI: Front Panel State >> Open"  # UI: Initialize UI: Front Panel State >> Open
            # "Initialization Macro\n(This is called once, when the VI starts)"
            n79 = call <vilib>:"Add State(s) to Queue__JKI_lib_State_Machine.vi"("State(s) in Front (\"\")"="Data: Initialize\nInitialize Core Data\nEvents: Register", "State(s) in (\"\")"="Process: Sync", "State(s) at Back (\"\")"=w244) -> ("States Out"=w243:string)  [unwired: 12 in]
            n80 = call <vilib>:"Add State(s) to Queue__jki_lib_state_machine.vi"("State(s) in Front (\"\")"=w243, "State(s) in (\"\")"=w250) -> ("States Out"=w249:string)  [unwired: 13 in]
          }
          frame "Macro: Exit" {
            # "Exit Macro\n(This is called once, when the VI exits)"
            n81 = Unbundle By Name(w255) -> ("Core.Close Panel on Exit?"=w261:bool)
            n82 = Select(t="UI: Front Panel State >> Close", s=w261, f="") -> (s? t:f=w258:string)
            n83 = call <vilib>:"Add State(s) to Queue__JKI_lib_State_Machine.vi"("State(s) in Front (\"\")"="Data: Cleanup\nEvents: Unregister", "State(s) in (\"\")"="Process: Sync", "State(s) at Back (\"\")"="Exit") -> ("States Out"=w252:string)  [unwired: 12 in]
            n84 = call <vilib>:"Add State(s) to Queue__jki_lib_state_machine.vi"("State(s) in (\"\")"=w258, "State(s) at Back (\"\")"=w252) -> ("States Out"=w257:string)  [unwired: 13 in]
            n85 = call <vilib>:"Add State(s) to Queue__jki_lib_state_machine.vi"("State(s) in Front (\"\")"=w257, "State(s) in (\"\")"=w264) -> ("States Out"=w263:string)  [unwired: 13 in]
          }
          frame "---------- Process ----------" {
            # "Template Separator\n(You can make a copy of, or modify, this frame)"
            n86 = call <vilib>:"Add State(s) to Queue__jki_lib_state_machine.vi"("State(s) in (\"\")"=w269) -> ("States Out"=w268:string)  [unwired: 14 in]
          }
          frame "Process: Sync" {
            n87 = Unbundle By Name(w277) -> ("Self Reference"=w273:refnum<class "Instrument.Example UI.lvclass">)
            n88 = call <vilib>:"WaitOnProcessSync.vi"("error in (no error)"=w272, "SMO"=w273) -> ("error out"=w271:errorcluster, "Don't run?"=w276:bool)  [unwired: 7 in, 1 out]
            n89 = Select(t="Data: Cleanup\nEvents: Unregister\nExit", s=w276, f="") -> (s? t:f=w270:string)
            n90 = call <vilib>:"Add State(s) to Queue__jki_lib_state_machine.vi"("State(s) in Front (\"\")"=w270, "State(s) in (\"\")"=w280) -> ("States Out"=w279:string)  [unwired: 13 in]
          }
          frame "Process: Self Terminate" {
            n91 = Unbundle By Name(w282) -> ("Self Reference"=w281:refnum<class "Instrument.Example UI.lvclass">)
            n92 = call <vilib>:"SelfTerminate.vi"("error in (no error)"=w284, "SMO in"=w281) -> ("error out"=w283:errorcluster)  [unwired: 8 in, 1 out]
            n93 = call <vilib>:"Add State(s) to Queue__jki_lib_state_machine.vi"("State(s) in (\"\")"=w287) -> ("States Out"=w286:string)  [unwired: 14 in]
          }
          frame "---------- Events ----------" {
            # "Template Separator\n(You can make a copy of, or modify, this frame)"
            n94 = call <vilib>:"Add State(s) to Queue__jki_lib_state_machine.vi"("State(s) in (\"\")"=w292) -> ("States Out"=w291:string)  [unwired: 14 in]
          }
          frame "Events: Register" {
            # "Expand to add\nmore events"
            # "Base Class Protected Events"
            n95 = Unbundle By Name(w303) -> ("Self Reference"=w296:refnum<class "Instrument.Example UI.lvclass">, "Instrument"=w295:refnum<class "Instrument.lvclass">)
            n96 = call <vilib>:"GetProtectedEvents.vi"("SMO"=w296) -> ("error out"=w297:errorcluster, "SMO Protected Events"=w301:T6)  [unwired: 8 in, 1 out]
            n97 = call <userlib>:"Instrument.GetPublicEvents.vi"("Instrument"=w295) -> ("error out"=w293:errorcluster, "Instrument Public Events"=w294:T7)  [unwired: 8 in, 1 out]
            n98 = register-events(w301, w294) -> (reference out=w302:refnum<event-registration>, error out=w299:errorcluster)  [unwired: 2 in]
            n99 = Merge Errors(w293, w300, w299, w297) -> (w298:errorcluster)
            n100 = call <vilib>:"Add State(s) to Queue__jki_lib_state_machine.vi"("State(s) in (\"\")"=w305) -> ("States Out"=w304:string)  [unwired: 14 in]
          }
          frame "Events: Unregister" {
            n101 = Unregister For Events(event registration refnum=w308, error in=w307) -> (error out=w306:errorcluster)
            n102 = call <vilib>:"Add State(s) to Queue__jki_lib_state_machine.vi"("State(s) in (\"\")"=w311) -> ("States Out"=w310:string)  [unwired: 14 in]
          }
          frame "---------- Action ----------" {
            n103 = Unbundle By Name(w314) -> ("Self Reference"=w312:refnum<class "Instrument.Example UI.lvclass">)
            n104 = Bundle By Name(cluster=w314, "Self Reference"=w312) -> (w313:T4)
            n105 = call <vilib>:"Add State(s) to Queue__jki_lib_state_machine.vi"("State(s) in (\"\")"=w318) -> ("States Out"=w317:string)  [unwired: 14 in]
          }
          frame "Action: Notify UI Closed" {
            # "Notify that the UI has been closed"
            n106 = Unbundle By Name(w321) -> ("Self Reference"=w322:refnum<class "Instrument.Example UI.lvclass">)
            n107 = call <vilib>:"Hide.vi"("error in (no error)"=w320, "SMO.UI"=w322) -> ("error out"=w319:errorcluster)  [unwired: 8 in, 1 out]
            n108 = call <vilib>:"Add State(s) to Queue__jki_lib_state_machine.vi"("State(s) in (\"\")"=w325) -> ("States Out"=w324:string)  [unwired: 14 in]
          }
          frame "Action: Update Front Panel All" {
            # "#todo\nyou must know data type of \"getAll\" and other commands"
            # "#todo\nprocess variant data like this"
            n109 = Unbundle By Name(w330) -> ("getAll"=w327:variant)
            n110 = Variant To Data(error in=w329, type=dbl[] [], Variant=w327) -> (error out=w328:errorcluster)  [unwired: 1 out]
            n111 = call <vilib>:"Add State(s) to Queue__jki_lib_state_machine.vi"("State(s) in (\"\")"=w333) -> ("States Out"=w332:string)  [unwired: 14 in]
          }
          frame "Action: Config" {
            # "#todo\nthis is configured to call Instrument.MessageToProcess.vi\nBut you could open a connection through STM and this can be a\nremote UI that runs from any machine (no examples are provided here\nyet (2/4/2019))"
            n112 = Unbundle By Name(w339) -> ("Instrument"=w338:refnum<class "Instrument.lvclass">, "config"=w336:variant)
            n113 = call <userlib>:"Instrument.MessageToProcess.vi"("error in (no error)"=w335, "Message.Data"=w336, "Message.Command"=w334, "Instrument"=w338) -> ("error out"=w337:errorcluster)  [unwired: 6 in, 1 out]
            n114 = call <vilib>:"Add State(s) to Queue__jki_lib_state_machine.vi"("State(s) in (\"\")"=w342) -> ("States Out"=w341:string)  [unwired: 14 in]
          }
        }
      }
    }
    frame Error {
    }
  }
  n115 = call-parent "Process.vi"("error in (no error)"=w8, "SMO.UI"=w7) -> ("error out"=w5:errorcluster, "SMO.UI out"=→"Example Instrument UI out":refnum<class "Instrument.Example UI.lvclass">)  [unwired: 8 in]
  n116 = Merge Errors(w5, w4) -> (→"error out":errorcluster)
